vi "Reset All Data.vi"(9 "Board Size":i32, 11 "AntFarm_MB":refnum<class "AntFarm_MB.lvclass">) -> (3 "AntFarm_MB Out":refnum<class "AntFarm_MB.lvclass">)   [LabVIEW 2016, in "AntFarm_MB.lvclass"]
uses:
  AntFarm_MB.lvclass
  TypeDefs/Cluster_Ant Farm Global Data.ctl
  Type Defs/Direction Enum.ctl
  AntFarm_MB.lvclass/AntFarm_MB.ctl
  Type Defs/SB Type Defs.lvlib
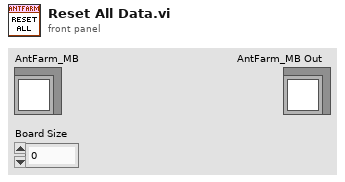
[diagram p1: front panel]
types:
  T1 = typedef "SB Type Defs.lvlib/Direction Enum.ctl" = enum16{"NW", "N", "NE", "E", "SE", "S", "SW", "W"}
  T2 = typedef "Cluster_Ant Farm Global Data.ctl" = cluster{"Move Map":i32[][], "Danger Map":i32[][], "Attack Rows":i32[], "Attack Columns":i32[], "Square count":i32, "Last Round":i32, "Danger Threshold":i32}
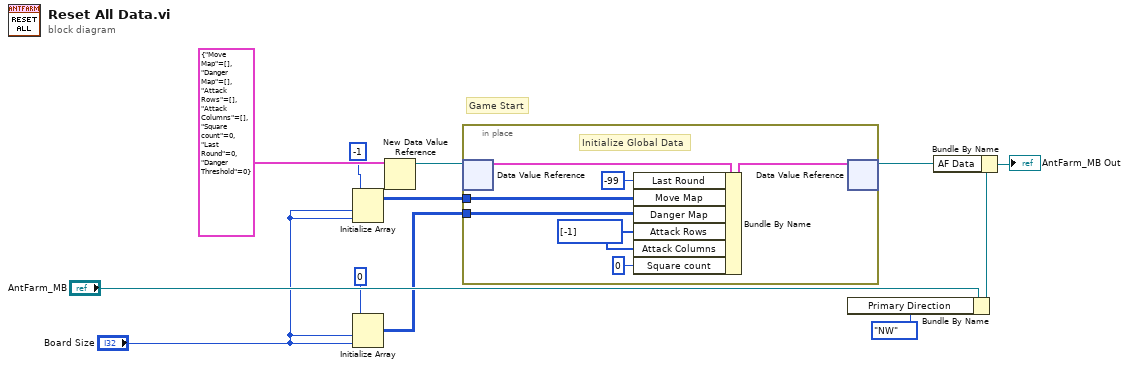
[diagram p0: block diagram]
diagram:
  # "Game Start"
  n1 = Initialize Array(-1 ("Round"), "Board Size", "Board Size") -> (w5:i32[][])
  n2 = Initialize Array(0 ("Round"), "Board Size", "Board Size") -> (w1:i32[][])
  n3 = New Data Value Reference(data value=T2 {"Move Map"=[], "Danger Map"=[], "Attack Rows"=[], "Attack Columns"=[], "Square count"=0, "Last Round"=0, "Danger Threshold"=0} ("Global Data")) -> (data value reference=w4:refnum<data-value>)  [unwired: 1 in, 1 out]
  n4 = in-place {
    in-place-border: w5 -> [w17]
    in-place-border: w1 -> [w16]
    w13 = i32[] [-1] ("Danger Rows")
    # "Initialize Global Data"
    n5 = in-place-dvr #1(w4) -> (w19:T2)  [unwired: 1 out]
    n6 = Bundle By Name(cluster=w19, "Last Round"=-99, "Move Map"=w17, "Danger Map"=w16, "Attack Rows"=w13, "Attack Columns"=w13, "Square count"=0) -> (w18:T2)
    n7 = in-place-dvr #1(w18) -> (w6:refnum<data-value>)  [unwired: 1 out]
  }
  n8 = Bundle By Name(cluster="AntFarm_MB", "Primary Direction"=Direction_Enum."NW" ("Data.Primary Direction")) -> (w2:refnum<class "AntFarm_MB.lvclass">)
  n9 = Bundle By Name(cluster=w2, "AF Data"=w6) -> (→"AntFarm_MB Out":refnum<class "AntFarm_MB.lvclass">)
